vi "LabVIEWRTControlStartupVI.vi"() -> ()   [LabVIEW 2014]
doc: "This example demonstrates a command based communication architecture using TCP. It shows a protocol for packaging and parsing data while minimizing network traffic. Refer to the National Instruments Web site at ni.com/info and enter the info code \"commtcp\" for more information about this command based communication architecture."
uses:
  Control 2.ctl
  ChannelCommand.ctl
  Control 1.ctl
  WaveType.ctl
  MoterEnable.ctl
  <userlib>/VMIC/VMIC 5565 Reflective Memory.llb/VMIC Reference.ctl
  <vilib>/Platform/TimedLoop/XDataNode/timing_clust.ctl
  <vilib>/Platform/TimedLoop/XDataNode/nitl_modes.ctl
  <vilib>/Platform/TimedLoop/XDataNode/wakeup.ctl
  <vilib>/DAQmx/write.llb/DAQmx Write (Analog 1D DBL NChan 1Samp).vi
  <userlib>/VMIC/VMIC 5565 Reflective Memory.llb/VMIC Write (U32).vi
  <vilib>/DAQmx/write.llb/DAQmx Write (Digital 1D Bool NChan 1Samp 1Line).vi
  <userlib>/VMIC/VMIC 5565 Reflective Memory.llb/VMIC Read (U8).vi
  <vilib>/Platform/TimedLoop/XDataNode/XDataNode.xnode
  <vilib>/Platform/TimedLoop/XDataNode/XDNodeRunTimeDep.lvlib
  <vilib>/real-time/NI_Real-Time Libraries.lvlib
  <vilib>/NI_Real-Time Target Support.lvlib
  <vilib>/real-time/rtutility.llb/RT Restart Target (Self).vi
panel:
  out "上传数组":dbl[](array[numeric])
  out "VMIC write":sgl[](array[numeric])
  out "6612counterTask 8":refnum<k21>
  out "6612counterTask 7":refnum<k21>
  out "6612counterTask 6":refnum<k21>
  out "6612counterTask 5":refnum<k21>
  out "当前时间":timestamp
  out "ResetAforce":dbl[](array[numeric])
  out "x/y":dbl
  out "全局结束时间":i64
  out "实际结束[i-1]":i64
  out "延迟完成？[i-1]":bool
  out "超时":i32=-1
  out "6612counterTask 4":refnum<k21>
  out "6612counterTask 3":refnum<k21>
  out "6612counterTask 2":refnum<k21> caption="任务输出"
  out "6612counterTask":refnum<k21>
  out "x与y? 4":bool[](array[boolean])
  out "x与y? 3":bool[](array[boolean])
  out "x与y? 2":bool[](array[boolean])
  out "VMIC reference":T1
  out "PXI6363IO":refnum<k21>
  out "x与y?":bool[](array[boolean])
  out "temp 8":bool
  out "temp 7":bool
  out "temp 6":bool
  out "temp 5":bool
  out "error out 6":errorcluster caption="error out"
  out "error out 4":errorcluster
  out "OutPut":dbl[](array[numeric])
  out "Command Type":i32
  out "Msg Head":string
  out "error out":errorcluster caption="错误输出"
  out "长度 3":i32
  out "长度 2":i32
  out "长度":i32
  out "connection ID":refnum<k5> caption="连接ID"
  out "6363Task":refnum<k21> caption="任务输出"
  out "error out 3":errorcluster caption="错误输出"
  out "加速度信号":dbl[](array[numeric])
  out "同步信号":dbl[](array[numeric])
  out "轴向位移":dbl[](array[numeric])
  out "轴向力":dbl[](array[numeric])
  out "T_outrange":bool[](array[boolean])
  out "error out 8":errorcluster caption="error out"
  out "error out 7":errorcluster caption="error out"
  out "error out 5":errorcluster caption="错误输出"
  out "diff syn out 2":dbl[](array[numeric])
  out "Forward":dbl[](array[numeric])
  out "AngleSampleData 2":dbl[](array[numeric])
  out "TorqueSampledata 2":dbl[](array[numeric])
  out "control out":dbl[](array[numeric])
  out "command out 2":dbl[](array[numeric])
  out "Wave out 2":dbl[](array[numeric])
  out "type out":dbl[](array[numeric])
  out "Enable":bool[](array[boolean])
  out "temp 4":bool
  out "temp 3":bool
  out "temp 2":bool
  out "temp 1":bool
  out "syn out":dbl[](array[numeric])
  out "TempAnOut":dbl[](array[numeric])
  out "StartChannelReset":bool[](array[boolean])
  out "retorquedata2":dbl[](array[numeric])
  out "reangeldata2":dbl[](array[numeric])
  out "output 4":dbl[](array[numeric])
  out "TestLoops 2":i32
  out "ResetAngle":dbl[](array[numeric])
  out "ResetTorque":dbl[](array[numeric])
  out "error out 2":errorcluster
  in  "Exit":bool
  out "ControlPara":dbl[][](array[numeric])
  out "ChannelSetArray":T2 {"Enable" items=["不使能", "使能"]; "Wave" items=["0指令", "正弦波", "方波", "三角波", "常值", "波形数据", "白噪声", "正弦扫频", "梯度加载", "VMIC"]; "ChannelType" items=["标准波形跟踪"=1, "扫频测试"=2, "消除多余力"=3, "梯度加载"=4, "载荷谱跟踪"=5, "模拟输入跟踪"=9]; "ChannelStatus" items=["通道关", "位置通道", "加载通道"]}
  out "Stop":bool
  out "iCommand":i32
  out "TestLoops":i32
  out "dt":dbl
  out "PXI6733Task":refnum<k21>
  out "Data array":dbl[][](array[numeric])
  out "error  out":errorcluster
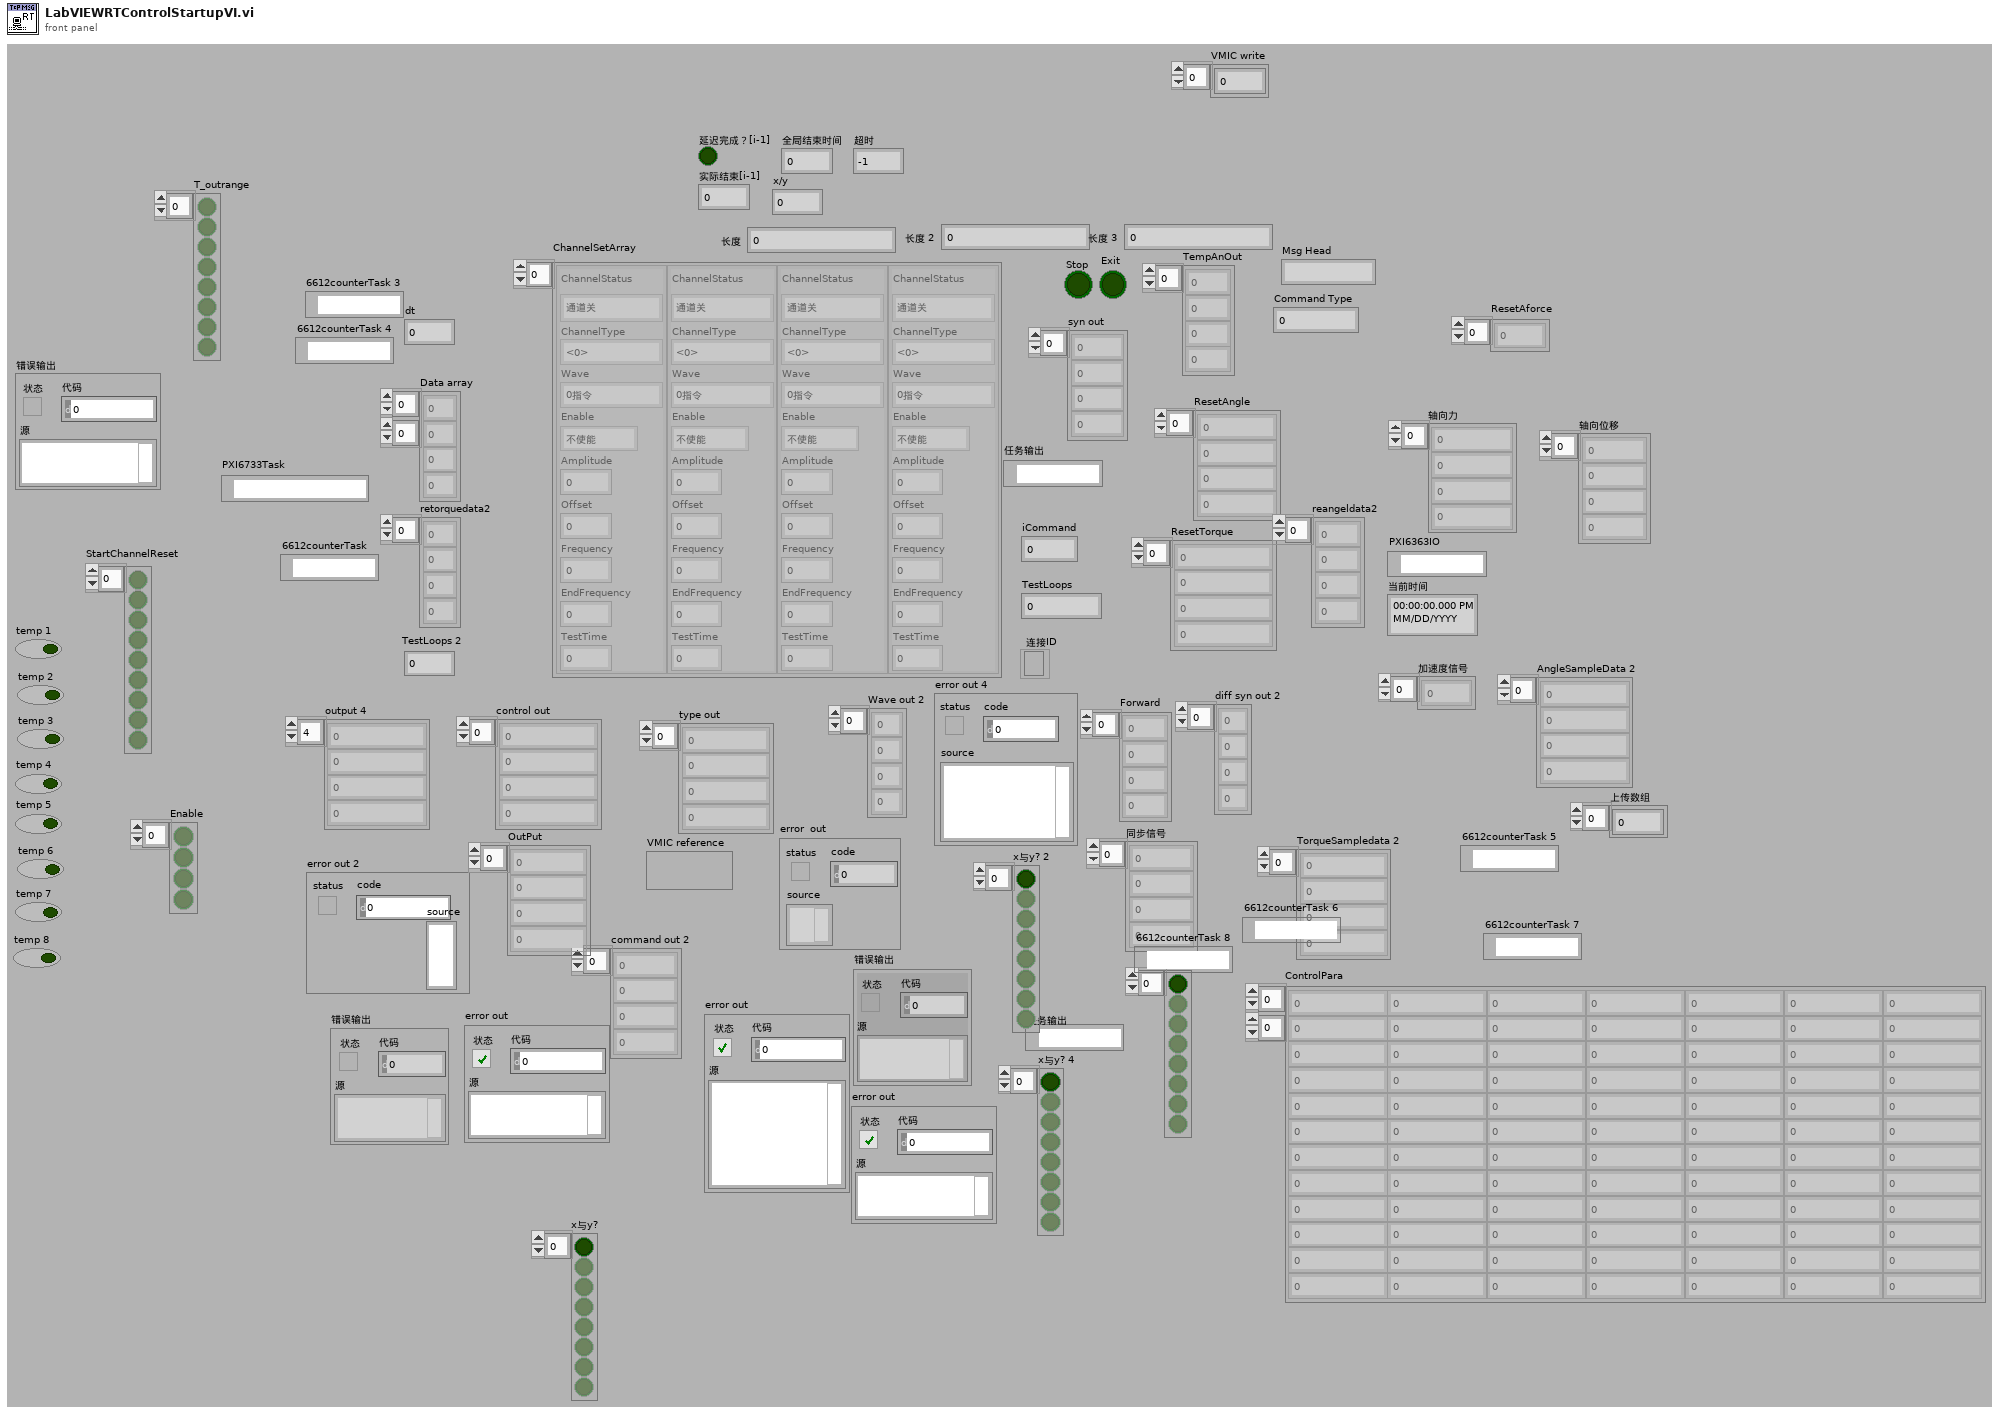
[diagram p1: front panel]
types:
  T1 = typedef "VMIC Reference.ctl" = variant
  T2 = typedef "Control 2.ctl" = T3[]
  T3 = typedef "ChannelCommand.ctl" = cluster{"ChannelStatus":T4, "ChannelType":i32, "Wave":T5, "Enable":T6, "Amplitude":dbl, "Offset":dbl, "Frequency":dbl, "EndFrequency":dbl, "TestTime":dbl}
  T4 = typedef "Control 1.ctl" = i32
  T5 = typedef "WaveType.ctl" = i32
  T6 = typedef "MoterEnable.ctl" = u16
  T7 = typedef "XDNodeRunTimeDep.lvlib/timing_clust.ctl" = cluster{"Expected End [f-1]":u64, "Actual End [f-1]":u64, "Finished Late? [f-1]":bool, "Expected End [i-1]":u64, "Actual End [i-1]":u64, "Finished Late? [i-1]":bool, "Expected Start [i]":u64, "Actual Start [i]":u64, "Expected Start [f]":u64, "Actual Start [f]":u64, "Source Name":string, "Structure Name":string, "Period":i64, "Deadline":i64, "Offset":i64, "Start":i64, "Priority":i32, "Timeout":i32, "Mode":T8, "Wakeup Reason":T9, "Error":errorcluster, "Source Type":string, "Secondary Source Type":string, "Global End Time":u64, "Global Start Time":u64, "Frame Duration":u64, "Iteration Duration":u64, "Assigned CPU":i32, "I/O Scan Engine Mode":u32}
  T8 = typedef "XDNodeRunTimeDep.lvlib/nitl_modes.ctl" = enum32{"No Change", "Process missed periods, maintain original phase", "Discard missed periods, maintain original phase", "Process missed periods, ignore original phase", "Discard missed periods, ignore original phase"}
  T9 = typedef "XDNodeRunTimeDep.lvlib/wakeup.ctl" = enum32{"Normal", "Aborted", "Asynchronous wakeup", "Timing source error", "Timed loop error", "Timeout"}
  T10 = enum16{"big-endian, network order", "native, host order", "little-endian"}
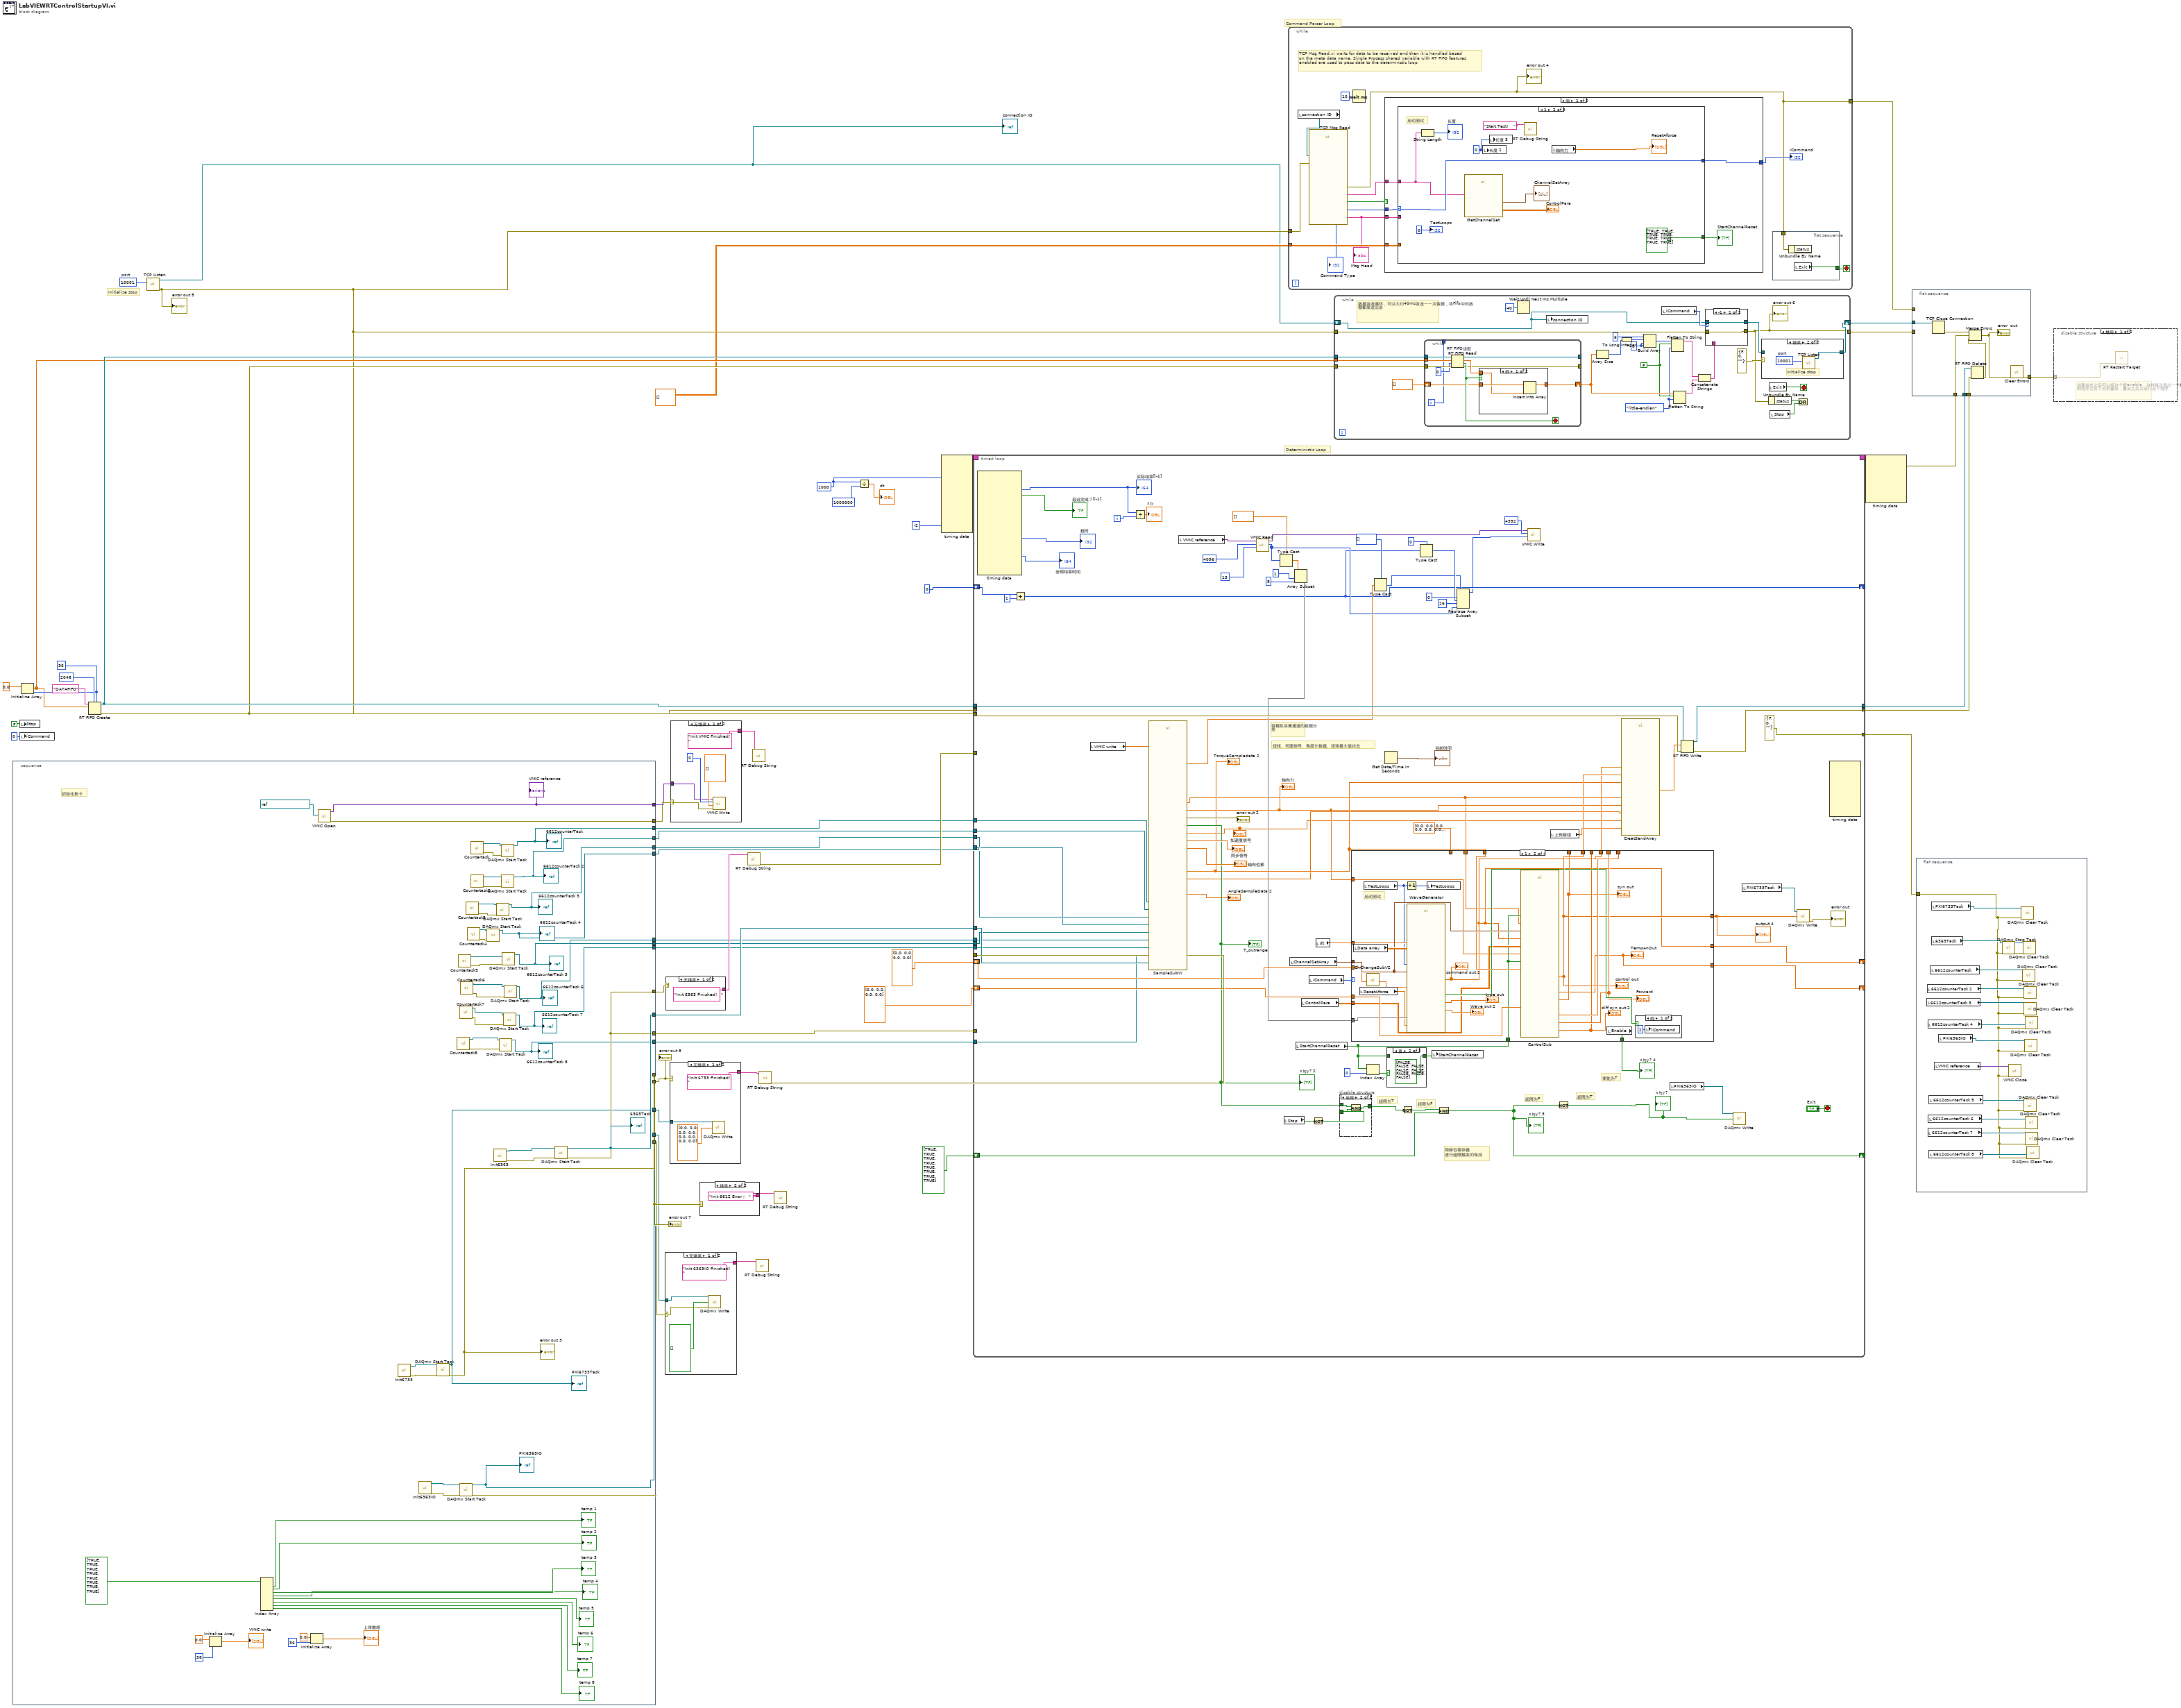
[diagram p0: block diagram]
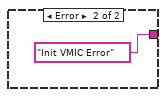
[diagram p2: hidden frame]
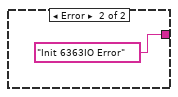
[diagram p3: hidden frame]
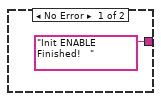
[diagram p4: hidden frame]
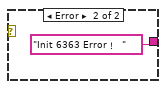
[diagram p5: hidden frame]
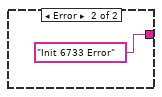
[diagram p7: hidden frame]
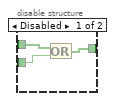
[diagram p8: hidden frame]
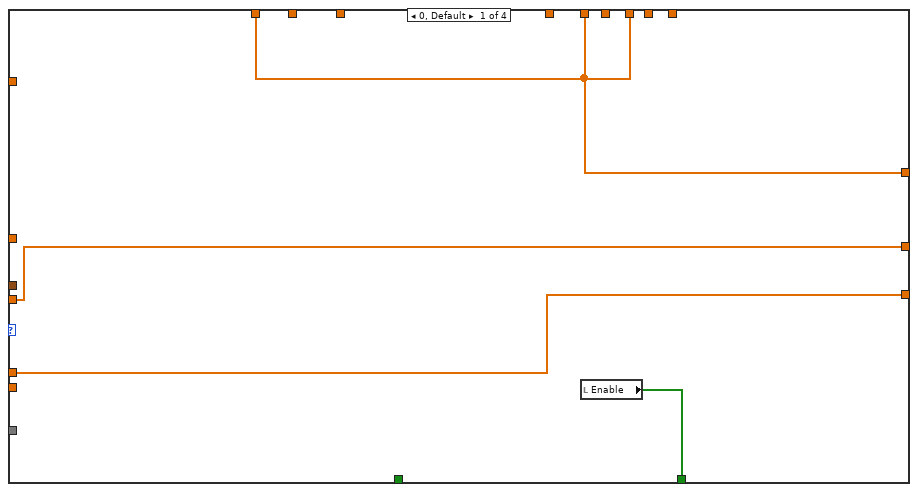
[diagram p10: hidden frame]
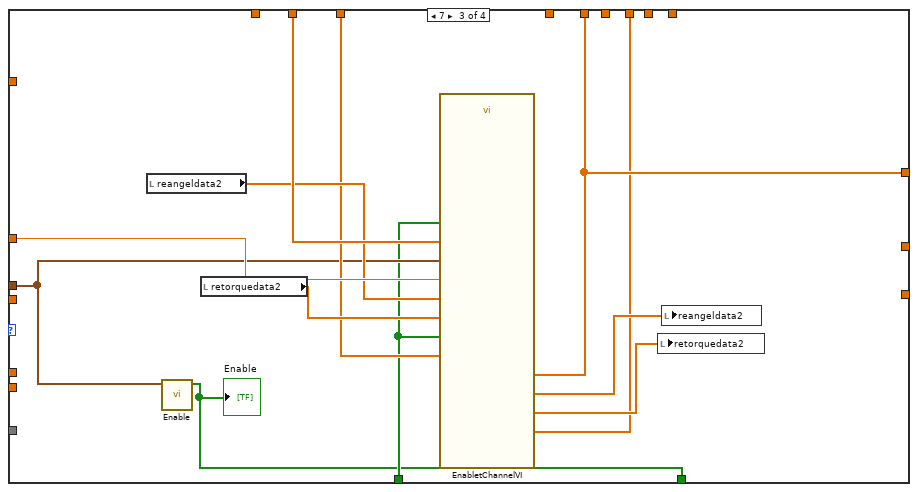
[diagram p12: hidden frame]
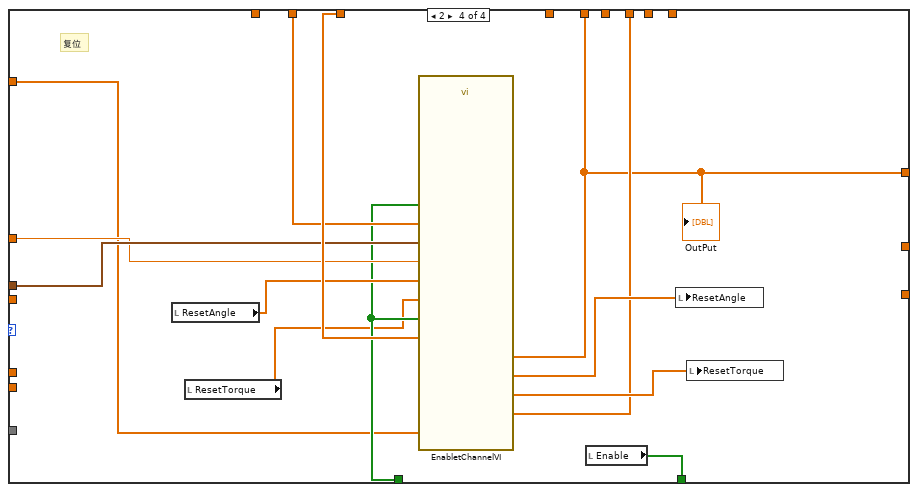
[diagram p13: hidden frame]
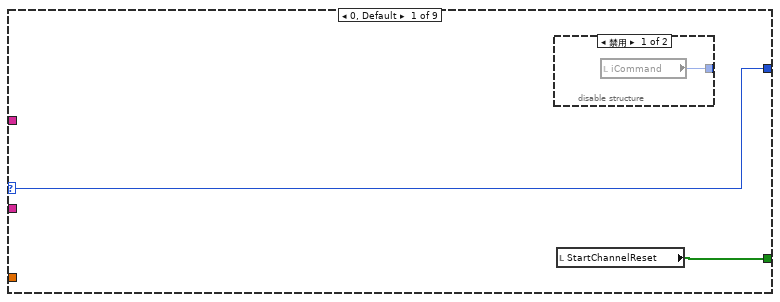
[diagram p14: hidden frame]
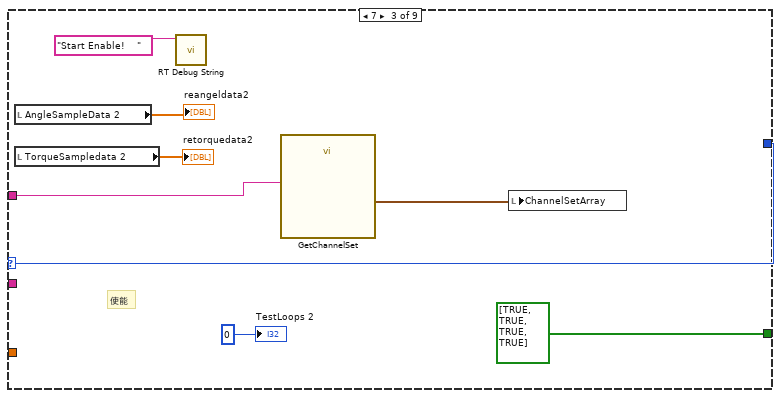
[diagram p16: hidden frame]
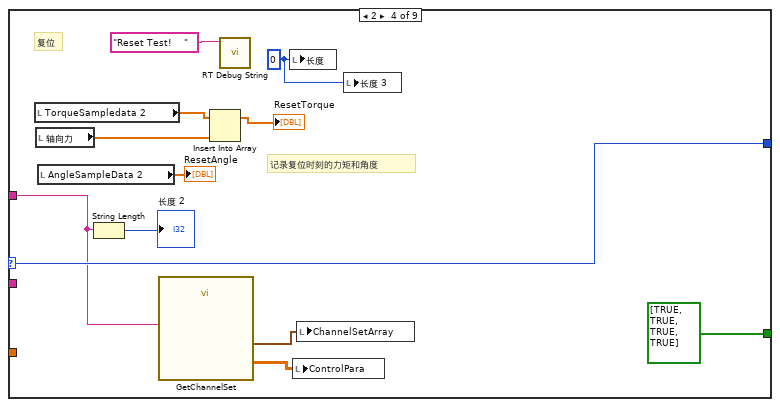
[diagram p17: hidden frame]
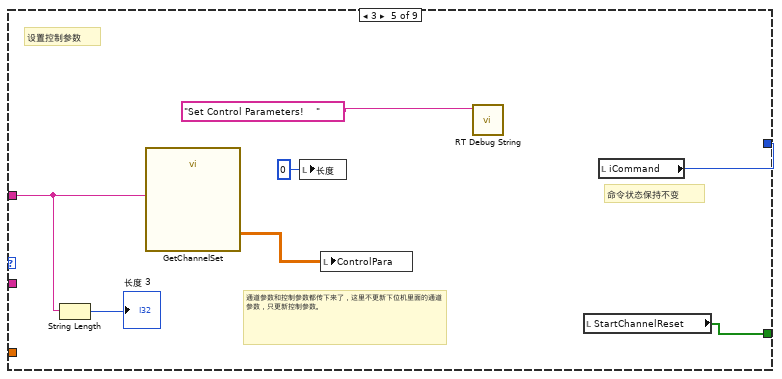
[diagram p18: hidden frame]
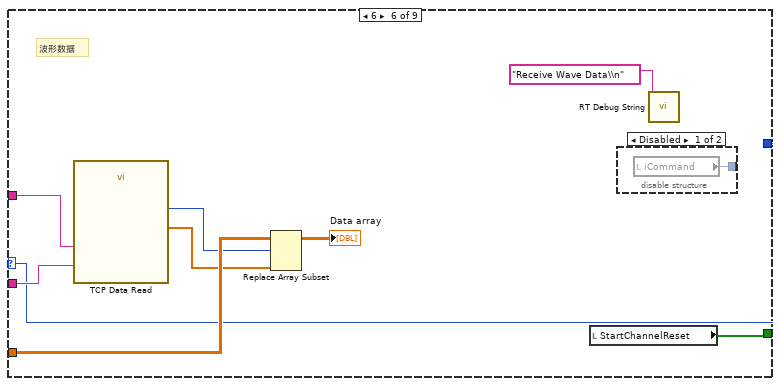
[diagram p19: hidden frame]
diagram:
  w44 = u32 36 ("elements in array (1)")
  w52 = i64 1000 ("Period")
  w56 = u16 10001  # port
  # "Deterministic Loop"
  # "Initialize stop"
  # "Command Parser Loop"
  n1 = stacked-sequence {
    tunnel: [w84] -> w23
    tunnel: [w84] -> w26
    tunnel: [w85] -> w22
    tunnel: [w82] -> w21
    tunnel: [w85] -> w7
    tunnel: [w86] -> w20
    tunnel: [w78] -> w15
    tunnel: [w80] -> w17
    tunnel: [w100] -> w14
    tunnel: [w99] -> w13
    tunnel: [w90] -> w11
    tunnel: [w89] -> w10
    tunnel: [w88] -> w9
    tunnel: [w87] -> w8
    tunnel: [w66] -> w6
    tunnel: [w65] -> w5
    tunnel: [w64] -> w4
    tunnel: [w63] -> w3
    frame #0 {
      # "初始化板卡"
      n2 = Initialize Array(sgl 0.0 ("元素"), 38 ("维数大小")) -> (→"VMIC write":sgl[])
      n3 = Index Array(array=bool[] [TRUE, TRUE, TRUE, TRUE, TRUE, TRUE, TRUE, TRUE] ("T_outrange 2")) -> (element #1=→"temp 1":bool, element #2=→"temp 2":bool, element #3=→"temp 3":bool, element #4=→"temp 4":bool, element #5=→"temp 5":bool, element #6=→"temp 6":bool, element #7=→"temp 7":bool, element #8=→"temp 8":bool)  [unwired: 8 in]
      n4 = Initialize Array(0.0 ("element"), 36 ("dimension size")) -> (→"上传数组":dbl[])
      n5 = call <userlib>:"VMIC Open.vi"("VISA resource name (empty)"=refnum<visa-resource-name> "PXI13::12::INSTR") -> ("error out"=w100:errorcluster, "VMIC reference"=w99:T1)  [unwired: 5 in]
      "VMIC reference" <- w99
      n6 = call "Init6733.vi"() -> ("error out"=w81:errorcluster, "task out"=w83:refnum<k21>)  [unwired: 10 in]
      n7 = call "Init6363IO.vi"() -> ("error out"=w77:errorcluster, "task out"=w79:refnum<k21>)  [unwired: 10 in]
      n8 = call <vilib>:"DAQmx Start Task.vi"("task/channels in"=w83, "error in"=w81) -> ("task out"=w82:refnum<k21>, "error out"=w84:errorcluster)  [unwired: 12 in]
      "PXI6733Task" <- w82
      "error out 3" <- w84
      n9 = call "Countertask8.vi"() -> ("error out"=w67:errorcluster, "task out"=w68:refnum<k21>)  [unwired: 10 in]
      n10 = call "Countertask5.vi"() -> ("error out"=w73:errorcluster, "task out"=w74:refnum<k21>)  [unwired: 10 in]
      n11 = call "Countertask7.vi"() -> ("error out"=w69:errorcluster, "task out"=w70:refnum<k21>)  [unwired: 10 in]
      n12 = call <vilib>:"DAQmx Start Task.vi"("task/channels in"=w79, "error in"=w77) -> ("task out"=w80:refnum<k21>, "error out"=w78:errorcluster)  [unwired: 12 in]
      "PXI6363IO" <- w80
      n13 = call "Countertask6.vi"() -> ("error out"=w71:errorcluster, "task out"=w72:refnum<k21>)  [unwired: 10 in]
      n14 = call "Countertask3.vi"() -> ("error out"=w93:errorcluster, "task out"=w94:refnum<k21>)  [unwired: 10 in]
      n15 = call "Countertask4.vi"() -> ("error out"=w91:errorcluster, "task out"=w92:refnum<k21>)  [unwired: 10 in]
      n16 = call "Countertask2.vi"() -> ("error out"=w95:errorcluster, "task out"=w96:refnum<k21>)  [unwired: 10 in]
      n17 = call "Countertask.vi"() -> ("error out"=w97:errorcluster, "task out"=w98:refnum<k21>)  [unwired: 10 in]
      n18 = call <vilib>:"DAQmx Start Task.vi"("task/channels in"=w92, "error in"=w91) -> ("task out"=w87:refnum<k21>)  [unwired: 12 in, 1 out]
      "6612counterTask 4" <- w87
      n19 = call "Init6363.vi"() -> ("error out"=w75:errorcluster, "task out"=w76:refnum<k21>)  [unwired: 10 in]
      n20 = call <vilib>:"DAQmx Start Task.vi"("task/channels in"=w94, "error in"=w93) -> ("task out"=w88:refnum<k21>)  [unwired: 12 in, 1 out]
      "6612counterTask 3" <- w88
      n21 = call <vilib>:"DAQmx Start Task.vi"("task/channels in"=w68, "error in"=w67) -> ("task out"=w63:refnum<k21>)  [unwired: 12 in, 1 out]
      "6612counterTask 8" <- w63
      n22 = call <vilib>:"DAQmx Start Task.vi"("task/channels in"=w98, "error in"=w97) -> ("task out"=w90:refnum<k21>)  [unwired: 12 in, 1 out]
      "6612counterTask" <- w90
      n23 = call <vilib>:"DAQmx Start Task.vi"("task/channels in"=w96, "error in"=w95) -> ("task out"=w89:refnum<k21>)  [unwired: 12 in, 1 out]
      "6612counterTask 2" <- w89
      n24 = call <vilib>:"DAQmx Start Task.vi"("task/channels in"=w74, "error in"=w73) -> ("task out"=w66:refnum<k21>)  [unwired: 12 in, 1 out]
      "6612counterTask 5" <- w66
      n25 = call <vilib>:"DAQmx Start Task.vi"("task/channels in"=w70, "error in"=w69) -> ("task out"=w64:refnum<k21>)  [unwired: 12 in, 1 out]
      "6612counterTask 7" <- w64
      n26 = call <vilib>:"DAQmx Start Task.vi"("task/channels in"=w72, "error in"=w71) -> ("task out"=w65:refnum<k21>)  [unwired: 12 in, 1 out]
      "6612counterTask 6" <- w65
      n27 = call <vilib>:"DAQmx Start Task.vi"("task/channels in"=w76, "error in"=w75) -> ("task out"=w86:refnum<k21>, "error out"=w85:errorcluster)  [unwired: 12 in]
      "6363Task" <- w86
    }
  }
  "error out 7" <- w26
  "error out 8" <- w23
  n28 = local write "Stop"(FALSE ("stop")) -> ()
  n29 = local write "iCommand"(0 ("iCommand")) -> ()
  n30 = Initialize Array(0.0, w44) -> (w43:dbl[])
  n31 = RT FIFO Create(0:"DATAFIFO" ("name (unnamed)"), 1:w43, 4:u32 2048 ("size (10)"), 6:w44) -> (8:w47:refnum<k33>, 11:w46:errorcluster)  [unwired: 4 in, 1 out]
  n32 = call <vilib>:"TCP Listen.vi"("port"=w56) -> ("error out"=w36:errorcluster, "connection ID"=w19:refnum<k5>)  [unwired: 3 in, 6 out]
  "error out 5" <- w36
  "connection ID" <- w19
  n33 = case shown="无错误" w15 {
    selector: w15 -> [w111 _]
    tunnel: ["Init 6363IO Finished!   " ("String to write") "Init 6363IO Error" ("String to write")] -> w16
    tunnel: w17 -> [w113 _]
    frame No Error {
      n34 = call-poly <vilib>:"DAQmx Write.vi"("task/channels in"=w113, "data"=bool[] [], "error in"=w111) -> ()  [unwired: 10 in, 3 out]
    }
    frame Error {
    }
  }
  n35 = case shown="无错误" w22 {
    tunnel: ["Init 6363 Finished!   " ("String to write") "Init 6363 Error！  " ("String to write")] -> w35
    frame No Error {
    }
    frame Error {
    }
  }
  n36 = case shown="无错误" w23 {
    tunnel: ["Init 6733 Finished!   " ("String to write") "Init 6733 Error" ("String to write")] -> w32
    tunnel: w21 -> [w118 _]
    frame No Error {
      n37 = call-poly <vilib>:"DAQmx Write.vi"("task/channels in"=w118, "data"=dbl[] [0.0, 0.0, 0.0, 0.0, 0.0, 0.0, 0.0, 0.0]) -> ()  [unwired: 11 in, 3 out]
    }
    frame Error {
    }
  }
  n38 = case shown="无错误" w14 {
    selector: w14 -> [w125 _]
    tunnel: ["Init VMIC Finished!   " ("String to write") "Init VMIC Error" ("String to write")] -> w12
    tunnel: w13 -> [w122 _]
    frame No Error {
      n39 = call-poly <userlib>:"VMIC Write.vi"("error in (no error)"=w125, "buffer"=dbl[] [], "offset (0)"=u32 0, "VMIC reference in"=w122) -> ()  [unwired: 2 in, 2 out]
    }
    frame Error {
    }
  }
  n40 = case shown="错误" w26 {
    tunnel: ["Init ENABLE Finished!   " ("String to write") "Init 6612 Error！  " ("String to write")] -> w27
    frame No Error {
    }
    frame Error {
    }
  }
  n41 = call <vilib>:"RT Debug String.vi"("String to write"=w35) -> ("error out"=w34:errorcluster)  [unwired: 10 in]
  n42 = call <vilib>:"RT Debug String.vi"("String to write"=w12) -> ()  [unwired: 10 in, 1 out]
  n43 = call <vilib>:"RT Debug String.vi"("String to write"=w16) -> ()  [unwired: 10 in, 1 out]
  n44 = call <vilib>:"RT Debug String.vi"("String to write"=w32) -> ("error out"=w33:errorcluster)  [unwired: 10 in]
  n45 = call <vilib>:"RT Debug String.vi"("String to write"=w27) -> ()  [unwired: 10 in, 1 out]
  n46 = Divide(x=w52, y=i64 1000000) -> (x/y=→"dt":dbl)
  n47 = node-c288(-2 ("Processor"), w52) -> (w55:T7)  [unwired: 7 in, 1 out]
  n48 = timed-loop "Timed Loop" {
    timing: w55 -> [_]
    timing-out: [_] -> w54
    tunnel: w47 -> [w213]
    tunnel: w46 -> [w211]
    tunnel: [w212] -> w28
    tunnel: [w210] -> w29
    tunnel: [errorcluster {"status"=FALSE, "code"=0, "source"=""} ("error in")] -> w37
    tunnel: w36 -> [_]
    tunnel: w34 -> [_]
    tunnel: w33 -> [_]
    shift-right: [w160] -> _
    shift-left: dbl[] [0.0, 0.0, 0.0, 0.0] -> [w194]
    shift-right: [w193] -> _
    shift-left: dbl[] [0.0, 0.0, 0.0, 0.0] -> [w192]
    tunnel: w20 -> [w189]
    tunnel: w7 -> [_]
    shift-right: [w178] -> _
    shift-left: bool[] [TRUE, TRUE, TRUE, TRUE, TRUE, TRUE, TRUE, TRUE] -> [w182]
    tunnel: w11 -> [w175]
    tunnel: w10 -> [w174]
    tunnel: w9 -> [w173]
    tunnel: w8 -> [w172]
    tunnel: w6 -> [w164]
    tunnel: w5 -> [w163]
    tunnel: w4 -> [w162]
    tunnel: w3 -> [w161]
    shift-right: [w142] -> _
    shift-left: 0 -> [w156]
    i -> [w168]
    stop <- "Exit" stop-if-true
    # "用移位寄存器\n进行超限触发的保持"
    # "使能为T"
    # "超限为T"
    # "超限为F"
    # "超限为T"
    # "超限为F"
    # "扭矩、伺服信号、角度计数器、扭矩最大值状态"
    # "将模拟采集通道的数据分类"
    n49 = node-c288() -> (w169:i64, →"延迟完成？[i-1]":bool, →"超时":i32, →"全局结束时间":i64)  [unwired: 13 out]
    "实际结束[i-1]" <- w169
    n50 = Add(x=w156, y=1) -> (x+y=w142:i32)
    n51 = local read "VMIC write"() -> (w140:sgl[])
    n52 = Divide(x=w169, y=w168) -> (x/y=→"x/y":dbl)
    n53 = call "SampleSubVI.vi"("task out"=w189, "Courter 1"=w175, "Courter 4"=w172, "Courter 2"=w174, "数组"=w140, "Courter 3"=w173, "Courter 7"=w162, "Courter 5"=w164, "Courter 8"=w161, "Courter 6"=w163) -> ("轴向位移"=→"轴向位移":dbl[], "轴向力"=w158:dbl[], "vmic反馈数据"=w143:sgl[], "AngleSample"=w148:dbl[], "加速度信号"=w141:dbl[], "同步信号"=→"同步信号":dbl[], "AngleSample 2"=→"AngleSampleData 2":dbl[], "F_outrange"=w179:bool[], "error out"=→"error out 2":errorcluster, "PositionSampleData"=w147:dbl[], "TorqueSample"=w159:dbl[])  [unwired: 3 in, 4 out]
    "TorqueSampledata 2" <- w159
    "T_outrange" <- w179
    "轴向力" <- w158
    "加速度信号" <- w141
    "x与y? 2" <- w179
    n54 = local read "VMIC reference"() -> (w134:T1)
    n55 = call-poly <userlib>:"VMIC Read.vi"("length (0)"=u32 13, "offset (0)"=u32 4096, "VMIC reference in"=w134) -> ("buffer"=w149:u32[], "VMIC reference out"=w138:T1)  [unwired: 2 in, 1 out]
    n56 = Type Cast(type=sgl[] [], x=w149) -> (*(type *) &x=w130:sgl[])
    n57 = local read "Stop"() -> (w185:bool)
    n58 = local read "ChannelSetArray"() -> (w204:T2)
    n59 = Array Subset(array=w130, index=1 ("索引"), length=8 ("长度")) -> (w154:sgl[])
    n60 = local read "StartChannelReset"() -> (w196:bool[])
    n61 = local read "ControlPara"() -> (w202:dbl[][])
    n62 = local read "iCommand"() -> (w201:i32)
    n63 = Not(x=w185) -> (.not. x?=w184:bool)
    n64 = local read "dt"() -> (w203:dbl)
    n65 = disable-structure shown="启用" {
      disable-tunnel: w184 -> [w221 w224]
      disable-tunnel: w179 -> [w220 w223]
      disable-tunnel: [w219 w222] -> w181
      frame Disabled {
        n66 = Or(x=w220, y=w221) -> (x .or. y?=w219:bool[])
      }
      frame Enabled {
        n67 = And(x=w223, y=w224) -> (x .and. y?=w222:bool[])
      }
    }
    n68 = case shown="1" w201 {
      tunnel: [w229 w233 w259 w274] -> w195
      tunnel: [w229 w234 w261 w272] -> w209
      tunnel: dbl[] [0.0, 0.0, 0.0, 0.0, 0.0, 0.0, 0.0, 0.0] ("Command") -> [w229 _ _ _]
      tunnel: [w229 w234 w261 w272] -> w200
      tunnel: w147 -> [_ w232 w269 w279]
      tunnel: w159 -> [_ w253 w265 w280]
      tunnel: w204 -> [_ w254 w264 w278]
      tunnel: w203 -> [_ w240 w268 w277]
      tunnel: w202 -> [_ w242 _ _]
      tunnel: w196 -> [_ w239 w260 w275]
      tunnel: [w230 w252 w258 w273] -> w177
      tunnel: [_ w241 _ _] -> _
      tunnel: w194 -> [w227 w248 _ _]
      tunnel: [w227 w231 _ _] -> w160
      tunnel: [_ w247 _ _] -> _
      tunnel: [_ w246 _ _] -> _
      tunnel: [_ w243 _ _] -> _
      tunnel: [w228 w233 _ _] -> w193
      tunnel: w192 -> [w228 w245 _ _]
      tunnel: w158 -> [_ w236 _ w271]
      tunnel: w154 -> [_ w238 _ _]
      frame 0, Default {
        n69 = local read "Enable"() -> (w230:bool[])
      }
      frame 1 {
        # "启动测试"
        n70 = local read "Data array"() -> (w255:dbl[][])
        n71 = local read "ResetAforce"() -> (w235:dbl[])
        n72 = local read "TestLoops"() -> (w237:i32)
        n73 = call "ChChangeSubV2.vi"("data in"=w245) -> ("data out"=w244:dbl[])  [unwired: 10 in]
        n74 = Increment(x=w237) -> (x+1=w256:i32)
        n75 = call "WaveGenerator.vi"("TestLoops"=w237, "AxisForce"=w235, "dt"=w240, "Angle"=w244, "WaveDefineArray"=w254, "VMIC command"=w238, "Data array"=w255) -> ("type out"=→"type out":dbl[], "Boolean"=w251:bool, "Command"=w233:dbl[], "wave out 2"=→"Wave out 2":dbl[])  [unwired: 1 in]
        "command out 2" <- w233
        n76 = local write "TestLoops"(w256) -> ()
        n77 = call "ControlSub.vi"("AxisForceSample"=w236, "Command"=w233, "Angel"=w239, "AngleSample"=w232, "TorqueSample"=w253, "Torque"=w239, "TempAnIn"=w248, "ChannelSetArray"=w254, "ControlPara"=w242) -> ("diff syn out 2"=w243:dbl[], "syn out"=w241:dbl[], "ControlOutput"=w234:dbl[], "Forward"=w247:dbl[], "TempAnOut"=w231:dbl[], "control out"=w246:dbl[])  [unwired: 4 in, 1 out]
        "TempAnOut" <- w231
        "syn out" <- w241
        "control out" <- w234
        "Forward" <- w247
        "diff syn out 2" <- w243
        n78 = local read "Enable"() -> (w252:bool[])
        n79 = case shown="假" w251 {
          frame False {
            n80 = local write "iCommand"(2 ("iCommand")) -> ()
          }
          frame True {
          }
        }
      }
      frame 7 {
        n81 = local read "reangeldata2"() -> (w267:dbl[])
        n82 = call "Enable.vi"("ChannelSetArray2"=w264) -> ("Enable"=w258:bool[])  [unwired: 10 in]
        "Enable" <- w258
        n83 = local read "retorquedata2"() -> (w266:dbl[])
        n84 = call "EnabletChannelVI.vi"("Angelsample"=w269, "Angel"=w260, "dt"=w268, "Torquesample"=w265, "Torque"=w260, "ResetAngel"=w267, "ResetTorqueCommand"=w266, "ChannelSetArray"=w264) -> ("OutPut"=w261:dbl[], "resetAngel 2"=w262:dbl[], "ResetTorque 2"=w263:dbl[], "Commandout"=w259:dbl[])  [unwired: 4 in]
        n85 = local write "retorquedata2"(w263) -> ()
        n86 = local write "reangeldata2"(w262) -> ()
      }
      frame 2 {
        # "复位"
        n87 = local read "ResetAngle"() -> (w276:dbl[])
        n88 = local read "ResetTorque"() -> (w270:dbl[])
        n89 = call "EnabletChannelVI.vi"("Angelsample"=w279, "Angel"=w275, "dt"=w277, "Torquesample"=w280, "Torque"=w275, "ResetAngel"=w276, "ResetTorqueCommand"=w270, "ChannelSetArray"=w278, "AxisForceSample"=w271) -> ("OutPut"=w272:dbl[], "resetAngel 2"=w281:dbl[], "ResetTorque 2"=w282:dbl[], "Commandout"=w274:dbl[])  [unwired: 3 in]
        "OutPut" <- w272
        n90 = local read "Enable"() -> (w273:bool[])
        n91 = local write "ResetAngle"(w281) -> ()
        n92 = local write "ResetTorque"(w282) -> ()
      }
    }
    "output 4" <- w200
    "x与y? 4" <- w177
    n93 = Index Array(array=w196, index=0) -> (element=w199:bool)
    n94 = Type Cast(type=u32[] [], x=w143) -> (*(type *) &x=w145:u32[])
    n95 = Get Date/Time In Seconds() -> (seconds since 1Jan1904=→"当前时间":timestamp)
    n96 = case shown="真" w199 {
      tunnel: [w225 bool[] [FALSE, FALSE, FALSE, FALSE, FALSE, FALSE, FALSE, FALSE]] -> w197
      tunnel: w196 -> [w225 _]
      frame False {
      }
      frame True {
      }
    }
    n97 = Not(x=w181) -> (.not. x?=w180:bool[])
    n98 = Type Cast(type=u32 0, x=w142) -> (*(type *) &x=w151:u32)
    n99 = local write "StartChannelReset"(w197) -> ()
    n100 = And(x=w180, y=w182) -> (x .and. y?=w178:bool[])
    "x与y? 3" <- w178
    n101 = Replace Array Subset(array=w145, new element #1=w151, index #1=0 ("索引"), new element #2=w149, index #2=29 ("索引")) -> (w137:u32[])
    n102 = call-poly <userlib>:"VMIC Write.vi"("buffer"=w137, "offset (0)"=u32 4352, "VMIC reference in"=w138) -> ()  [unwired: 3 in, 2 out]
    n103 = local read "上传数组"() -> (w146:dbl[])
    n104 = Not(x=w178) -> (.not. x?=w176:bool[])
    "x与y?" <- w176
    n105 = call "CreatSendArray.vi"("AngleSample"=w148, "AxisForces"=w158, "AccumulateSample"=w141, "数组"=w146, "DisplacementSample"=w147, "ControlOutput"=w209, "TorqueSampledata"=w159, "Command"=w195) -> ("SendArray"=w208:dbl[])  [unwired: 3 in]
    n106 = local read "PXI6363IO"() -> (w183:refnum<k21>)
    n107 = RT FIFO Write(0:w213, 1:w208, 3:w211) -> (8:w212:refnum<k33>, 11:w210:errorcluster)  [unwired: 2 in, 2 out]
    n108 = call-poly <vilib>:"DAQmx Write.vi"("task/channels in"=w183, "data"=w176) -> ()  [unwired: 11 in, 3 out]
    n109 = local read "PXI6733Task"() -> (w186:refnum<k21>)
    n110 = call-poly <vilib>:"DAQmx Write.vi"("task/channels in"=w186, "data"=w200) -> ("error out"=→"error out":errorcluster)  [unwired: 11 in, 2 out]
    n111 = node-c288() -> ()  [unwired: 7 in, 2 out]
  }
  n112 = while {
    tunnel: w36 -> [w294]
    tunnel: [w287] -> w30
    tunnel: dbl[][] [] -> [w291]
    stop <- w286 stop-if-true
    # "TCP Msg Read.vi waits for data to be received and then it is handled based \non the meta data name. Single Process shared variable with RT FIFO features \nenabled are used to pass data to the determinstic loop"
    n113 = local read "connection ID"() -> (w284:refnum<k5>)
    n114 = call "TCP Msg Read.vi"("connection ID"=w284, "error in"=w294) -> ("Timed Out?"=w293:bool, "Command Type"=w289:i32, "Msg Data"=w292:string, "Msg Head"=w290:string, "error out"=w287:errorcluster)  [unwired: 12 in, 1 out]
    "Msg Head" <- w290
    "Command Type" <- w289
    "error out 4" <- w287
    n115 = Wait (ms)(milliseconds to wait=u32 10 ("等待时间（毫秒）")) -> ()  [unwired: 1 out]
    n116 = case shown="假" w293 {
      tunnel: w292 -> [w302 _]
      tunnel: w289 -> [w301 _]
      tunnel: w291 -> [w300 _]
      tunnel: w290 -> [w299 _]
      tunnel: [w298 w360] -> w288
      frame False {
        n117 = case shown="1" w301 {
          selector: w301 -> [w304 w311 w320 w333 _ w344 w354 w356 _]
          tunnel: w302 -> [_ w309 w323 w327 w337 w351 _ _ _]
          tunnel: w300 -> [_ _ _ _ _ w350 _ _ _]
          tunnel: w299 -> [_ _ _ _ _ w345 _ _ _]
          tunnel: [w304 w311 w320 w333 w340 w344 w354 w356 w359] -> w298
          tunnel: [w303 bool[] [TRUE, TRUE, TRUE, TRUE, TRUE, TRUE, TRUE, TRUE] bool[] [TRUE, TRUE, TRUE, TRUE] bool[] [TRUE, TRUE, TRUE, TRUE] w339 w343 w353 w355 w358] -> w297
          frame 0, Default {
            n118 = disable-structure shown="禁用" {
              disable-tunnel: [w305 _] -> _
              frame Disabled {
                n119 = local read "iCommand"() -> (w305:i32)
              }
              frame Enabled {
              }
            }
            n120 = local read "StartChannelReset"() -> (w303:bool[])
          }
          frame 1 {
            w307 = 0 ("长度 2")
            # "启动测试"
            n121 = String Length(string=w309) -> (length=→"长度":i32)
            n122 = call "GetChannelSet.vi"("Msg Data"=w309) -> ("ControlPara"=→"ControlPara":dbl[][], "ChannelSetArray"=→"ChannelSetArray":T3[])  [unwired: 9 in]
            n123 = local write "长度 2"(w307) -> ()
            n124 = local write "长度 3"(w307) -> ()
            n125 = call <vilib>:"RT Debug String.vi"("String to write"="Start Test!    ") -> ()  [unwired: 10 in, 1 out]
            n126 = local read "轴向力"() -> (→"ResetAforce":dbl[])
            "TestLoops" <- 0 ("TestLoops")
          }
          frame 7 {
            # "使能"
            n127 = local read "AngleSampleData 2"() -> (→"reangeldata2":dbl[])
            n128 = local read "TorqueSampledata 2"() -> (→"retorquedata2":dbl[])
            n129 = call <vilib>:"RT Debug String.vi"("String to write"="Start Enable!    ") -> ()  [unwired: 10 in, 1 out]
            n130 = call "GetChannelSet.vi"("Msg Data"=w323) -> ("ChannelSetArray"=w317:T3[])  [unwired: 9 in, 1 out]
            n131 = local write "ChannelSetArray"(w317) -> ()
            "TestLoops 2" <- 0 ("TestLoops")
          }
          frame 2 {
            w324 = 0 ("长度")
            # "记录复位时刻的力矩和角度"
            # "复位"
            n132 = local read "TorqueSampledata 2"() -> (w330:dbl[])
            n133 = local read "轴向力"() -> (w329:dbl[])
            n134 = local read "AngleSampleData 2"() -> (→"ResetAngle":dbl[])
            n135 = String Length(string=w327) -> (length=→"长度 2":i32)
            n136 = call "GetChannelSet.vi"("Msg Data"=w327) -> ("ControlPara"=w325:dbl[][], "ChannelSetArray"=w326:T3[])  [unwired: 9 in]
            n137 = Insert Into Array(array=w330, new element=w329) -> (→"ResetTorque":dbl[])  [unwired: 1 in]
            n138 = call <vilib>:"RT Debug String.vi"("String to write"="Reset Test!    ") -> ()  [unwired: 10 in, 1 out]
            n139 = local write "长度"(w324) -> ()
            n140 = local write "ControlPara"(w325) -> ()
            n141 = local write "ChannelSetArray"(w326) -> ()
            n142 = local write "长度 3"(w324) -> ()
          }
          frame 3 {
            # "命令状态保持不变"
            # "通道参数和控制参数都传下来了，这里不更新下位机里面的通道参数，只更新控制参数。"
            # "设置控制参数"
            n143 = String Length(string=w337) -> (length=→"长度 3":i32)
            n144 = call "GetChannelSet.vi"("Msg Data"=w337) -> ("ControlPara"=w342:dbl[][])  [unwired: 9 in, 1 out]
            n145 = local write "长度"(0 ("长度")) -> ()
            n146 = local write "ControlPara"(w342) -> ()
            n147 = call <vilib>:"RT Debug String.vi"("String to write"="Set Control Parameters!    ") -> ()  [unwired: 10 in, 1 out]
            n148 = local read "StartChannelReset"() -> (w339:bool[])
            n149 = local read "iCommand"() -> (w340:i32)
          }
          frame 6 {
            # "波形数据"
            n150 = call "TCP Data Read.vi"("Data"=w351, "Head"=w345) -> ("Data Channel"=w346:i32, "DataArray"=w349:dbl[])  [unwired: 8 in]
            n151 = Replace Array Subset(array=w350, new element=w349, index (row)=w346) -> (→"Data array":dbl[][])  [unwired: 1 in]
            n152 = local read "StartChannelReset"() -> (w343:bool[])
            n153 = disable-structure shown="Disabled" {
              disable-tunnel: [w352 _] -> _
              frame Disabled {
                n154 = local read "iCommand"() -> (w352:i32)
              }
              frame Enabled {
              }
            }
            n155 = call <vilib>:"RT Debug String.vi"("String to write"="Receive Wave Data\\n") -> ()  [unwired: 10 in, 1 out]
          }
          frame 4 {
            # "停止测试"
            n156 = local read "StartChannelReset"() -> (w353:bool[])
          }
          frame -1 {
            # "退出测试"
            n157 = local read "StartChannelReset"() -> (w355:bool[])
            "Stop" <- TRUE
          }
          frame 88 {
            # "看门狗指令"
            n158 = local read "StartChannelReset"() -> (w358:bool[])
            n159 = local read "iCommand"() -> (w359:i32)
          }
        }
        "StartChannelReset" <- w297
      }
      frame True {
        n160 = local read "iCommand"() -> (w360:i32)
      }
    }
    "iCommand" <- w288
    n161 = flat-sequence {
      tunnel: w287 -> [w296]
      tunnel: [w295] -> w286
      frame #0 {
        n162 = Unbundle By Name(w296) -> ()  [unwired: 1 out]
        n163 = local read "Exit"() -> (w295:bool)
      }
    }
  }
  n164 = while {
    tunnel: w36 -> [w384]
    tunnel: [w361] -> w31
    tunnel: w47 -> [w382]
    tunnel: w46 -> [w383]
    tunnel: w43 -> [w381]
    shift-right: [w364] -> w38
    shift-left: w19 -> [w363]
    stop <- w366 stop-if-true
    w369 = 0 ("element")
    w373 = FALSE ("prepend array or string size? (T)")
    w372 = T10."little-endian" ("byte order (0:big-endian, network order)")
    # "数据发送循环，可以大约40ms发送一一次数据，将Fifo中的数据都发送出去"
    n165 = while {
      tunnel: w382 -> [w407]
      tunnel: w383 -> [w406]
      tunnel: w381 -> [w405]
      shift-right: [w398] -> w377
      shift-left: dbl[] [] -> [w399]
      tunnel: [w403] -> _
      tunnel: [w400] -> _
      tunnel: [w397] -> _
      i -> [w397]
      stop <- w402 stop-if-true
      n166 = RT FIFO Read "RT FIFO读取"(0:w407, 1:w405, 2:0 ("timeout in ms (0)"), 3:w406) -> (8:w403:refnum<k33>, 9:w401:dbl[], 10:w402:bool, 11:w400:errorcluster)  [unwired: 1 out]
      n167 = case shown="假" w402 {
        tunnel: w401 -> [w408 _]
        tunnel: w399 -> [w410 w411]
        tunnel: [w409 w411] -> w398
        frame False {
          n168 = Insert Into Array(array=w410, new element=w408) -> (w409:dbl[])  [unwired: 1 in]
        }
        frame True {
        }
      }
    }
    n169 = Wait Until Next ms Multiple(millisecond multiple=u32 40) -> ()  [unwired: 1 out]
    n170 = local write "connection ID"(w363) -> ()
    n171 = Array Size(array=w377) -> (size(s)=w368:i32)
    n172 = To Long Integer(number=w368) -> (32bit integer=w370:i32)
    n173 = Build Array(6 ("data"), w370, w369, w369) -> (w374:i32[])
    n174 = local read "iCommand"() -> (w367:i32)
    n175 = Flatten To String(anything=w374, prepend array or string size? (T)=w373, byte order (0:big-endian, network order)=w372) -> (data string=w371:string)  [unwired: 1 in, 2 out]
    n176 = Flatten To String(anything=w377, prepend array or string size? (T)=w373, byte order (0:big-endian, network order)=w372) -> (data string=w376:string)  [unwired: 1 in, 2 out]
    n177 = Concatenate Strings(w371, w376) -> (w378:string)
    n178 = case shown="-1" w367 {
      tunnel: w363 -> [w391 w396]
      tunnel: [w391 w395] -> w365
      tunnel: [w390 w394] -> w361
      tunnel: w384 -> [w390 w393]
      tunnel: w378 -> [_ w392]
      frame -1 {
      }
      frame 0, Default {
        n179 = TCP Write(connection ID=w396, data in=w392, error in (no error)=w393) -> (connection ID out=w395:refnum<k5>, error out=w394:errorcluster)  [unwired: 1 in, 1 out]
      }
    }
    "error out 6" <- w361
    n180 = case shown="错误" errorcluster {"status"=FALSE, "code"=0, "source"=""} ("error IO") {
      tunnel: w365 -> [w387 _]
      tunnel: [w387 w388] -> w364
      frame No Error {
      }
      frame Error {
        w389 = u16 10001  # port
        # "Initialize stop"
        n181 = call <vilib>:"TCP Listen.vi"("port"=w389) -> ("connection ID"=w388:refnum<k5>)  [unwired: 3 in, 7 out]
      }
    }
    n182 = Unbundle By Name(w361) -> ("status"=w385:bool)
    n183 = local read "Exit"() -> (w366:bool)
    n184 = local read "Stop"() -> (w380:bool)
    n185 = Or(x=w385, y=w380) -> ()  [unwired: 1 out]
  }
  n186 = node-c288(w54) -> (w53:errorcluster)  [unwired: 5 out]
  n187 = flat-sequence {
    tunnel: w53 -> [w419]
    tunnel: [w418] -> w25
    tunnel: w38 -> [w417]
    tunnel: w31 -> [_]
    tunnel: w30 -> [_]
    tunnel: w29 -> [w414]
    tunnel: w28 -> [w413]
    frame #0 {
      n188 = TCP Close Connection(connection ID=w417) -> (error out=w416:errorcluster)  [unwired: 1 in, 2 out]
      n189 = RT FIFO Delete(0:w413, 3:w414) -> (11:w412:errorcluster)  [unwired: 1 in]
      n190 = Merge Errors(w416, w419, w412) -> (w415:errorcluster)
      "error  out" <- w415
      n191 = call <vilib>:"Clear Errors.vi"("error in (no error)"=w415) -> ("error out"=w418:errorcluster)  [unwired: 5 in, 1 out]
    }
  }
  n192 = flat-sequence {
    tunnel: w37 -> [w420]
    frame #0 {
      n193 = local read "6612counterTask 3"() -> (w428:refnum<k21>)
      n194 = local read "6612counterTask 2"() -> (w429:refnum<k21>)
      n195 = local read "6612counterTask 4"() -> (w427:refnum<k21>)
      n196 = local read "6612counterTask 7"() -> (w423:refnum<k21>)
      n197 = local read "6612counterTask 6"() -> (w422:refnum<k21>)
      n198 = local read "6612counterTask 5"() -> (w421:refnum<k21>)
      n199 = local read "6612counterTask 8"() -> (w424:refnum<k21>)
      n200 = local read "6612counterTask"() -> (w430:refnum<k21>)
      n201 = local read "PXI6733Task"() -> (w431:refnum<k21>)
      n202 = local read "6363Task"() -> (w432:refnum<k21>)
      n203 = local read "VMIC reference"() -> (w425:T1)
      n204 = local read "PXI6363IO"() -> (w426:refnum<k21>)
      n205 = call <vilib>:"DAQmx Stop Task.vi"("task/channels in"=w432, "error in"=w420) -> ("task out"=w434:refnum<k21>, "error out"=w433:errorcluster)  [unwired: 12 in]
      n206 = call <userlib>:"VMIC Close.vi"("error in (no error)"=w420, "VMIC reference in"=w425) -> ()  [unwired: 5 in, 1 out]
      n207 = call <vilib>:"DAQmx Clear Task.vi"("task in"=w431, "error in"=w420) -> ()  [unwired: 13 in, 1 out]
      n208 = call <vilib>:"DAQmx Clear Task.vi"("task in"=w430, "error in"=w420) -> ()  [unwired: 13 in, 1 out]
      n209 = call <vilib>:"DAQmx Clear Task.vi"("task in"=w434, "error in"=w433) -> ()  [unwired: 13 in, 1 out]
      n210 = call <vilib>:"DAQmx Clear Task.vi"("task in"=w421, "error in"=w420) -> ()  [unwired: 13 in, 1 out]
      n211 = call <vilib>:"DAQmx Clear Task.vi"("task in"=w429, "error in"=w420) -> ()  [unwired: 13 in, 1 out]
      n212 = call <vilib>:"DAQmx Clear Task.vi"("task in"=w428, "error in"=w420) -> ()  [unwired: 13 in, 1 out]
      n213 = call <vilib>:"DAQmx Clear Task.vi"("task in"=w426, "error in"=w420) -> ()  [unwired: 13 in, 1 out]
      n214 = call <vilib>:"DAQmx Clear Task.vi"("task in"=w427, "error in"=w420) -> ()  [unwired: 13 in, 1 out]
      n215 = call <vilib>:"DAQmx Clear Task.vi"("task in"=w422, "error in"=w420) -> ()  [unwired: 13 in, 1 out]
      n216 = call <vilib>:"DAQmx Clear Task.vi"("task in"=w423, "error in"=w420) -> ()  [unwired: 13 in, 1 out]
      n217 = call <vilib>:"DAQmx Clear Task.vi"("task in"=w424, "error in"=w420) -> ()  [unwired: 13 in, 1 out]
    }
  }
  n218 = disable-structure shown="禁用" {
    disable-tunnel: w25 -> [w435 _]
    frame Disabled {
      # "如果发布之后可以将这个框enable，这样每次退出一个控制程序之后下位机重启，重启之后又运行这个程序"
      n219 = call-poly <vilib>:"RT Restart Target.vi"("error in (no error)"=w435) -> ()  [unwired: 10 in, 1 out]
    }
    frame Enabled {
    }
  }
